vi "OpenConnection.vi"(8 "error in (no error)":errorcluster, 9 "Timeout (ms)":u32=5000 min=1, 10 "Connection Params":T1={"Vid"=0, "Pid"=0, "Device Index"=0, "u32_I2Cclk"=100} {"u32_I2Cclk" min=100 max=4000 step=1 format="%d Kbps"; "Pid" format="%.0x"; "Vid" format="%.0x"}, 11 "ProdType_1 in":refnum<class "ProdType_1.lvclass">) -> (0 "error out":errorcluster, 3 "ProdType_1 out":refnum<class "ProdType_1.lvclass">)   [LabVIEW 2020, in "I2COUSB.lvlib" / "ProdType_1.lvclass"]
doc: "Open connection"
uses:
  ProdType_1.lvclass
  II2COUSB/II2COUSB/ConnectionParams.ctl
  II2COUSB/II2COUSB/II2COUSB.lvclass
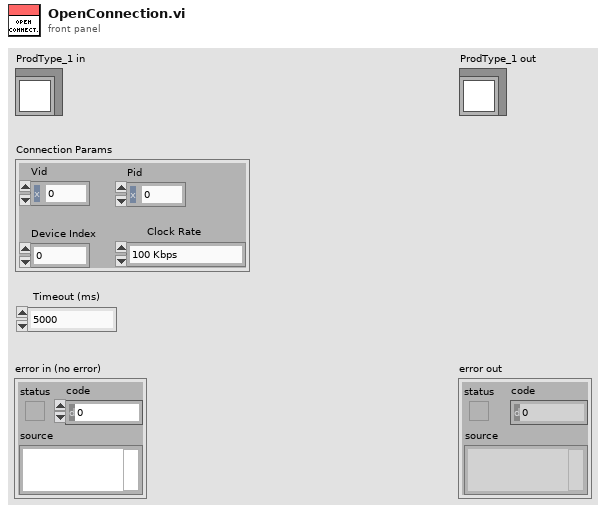
[diagram p1: front panel]
types:
  T1 = typedef "II2COUSB.lvlib/II2COUSB.lvclass/ConnectionParams.ctl" = cluster{"Vid":u16, "Pid":u16, "Device Index":u32, "u32_I2Cclk":u32}
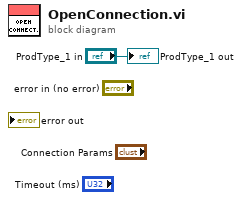
[diagram p0: block diagram]
diagram:
  "ProdType_1 out" <- "ProdType_1 in"
